vi "Write Dots.vi"(8 "error in (no error)":errorcluster, 10 "Dots":refnum<class "Dot Settings.lvclass">[](array[class]), 11 "Setting Database in":refnum<class "Setting Database.lvclass">) -> (0 "error out":errorcluster, 3 "Setting Database out":refnum<class "Setting Database.lvclass">)   [LabVIEW 2019, in "Setting Database.lvclass"]
uses:
  Setting Database.lvclass
  Dot Settings/Dot Settings.lvclass
  Setting Database.lvclass/Setting Database.ctl
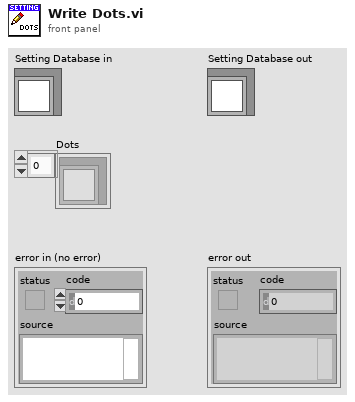
[diagram p1: front panel]
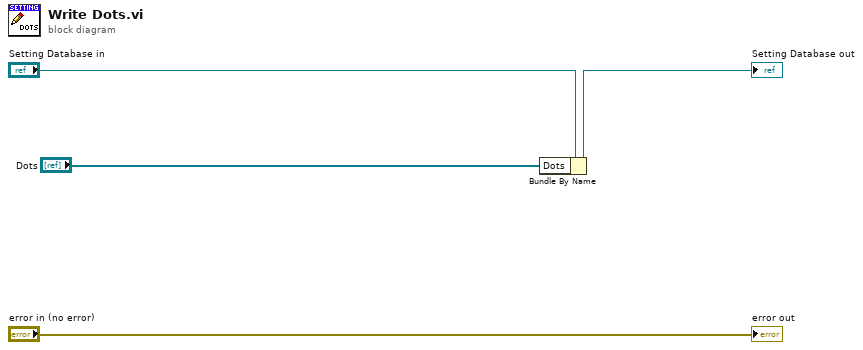
[diagram p0: block diagram]
diagram:
  n1 = Bundle By Name(cluster="Setting Database in", "Dots"="Dots") -> (→"Setting Database out":refnum<class "Setting Database.lvclass">)
  "error out" <- "error in (no error)"
